vi "Write to file.vi"(8 "error in (no error)":errorcluster, 9 "Data Cluster":T4, 10 "Test Case":T5, 11 "Don't wait for stabilizatoin":bool) -> (0 "error out":errorcluster)   [LabVIEW 2013]
uses:
  Controls/Test Case.ctl
  Controls/Power Values.ctl
  <vilib>/addons/Electrical Power/Basic/Measurement/subVIs/basic_Power Value.ctl
  Controls/Stabilization.ctl
  <vilib>/addons/Electrical Power/Basic/NI_EP_Basic.lvlib
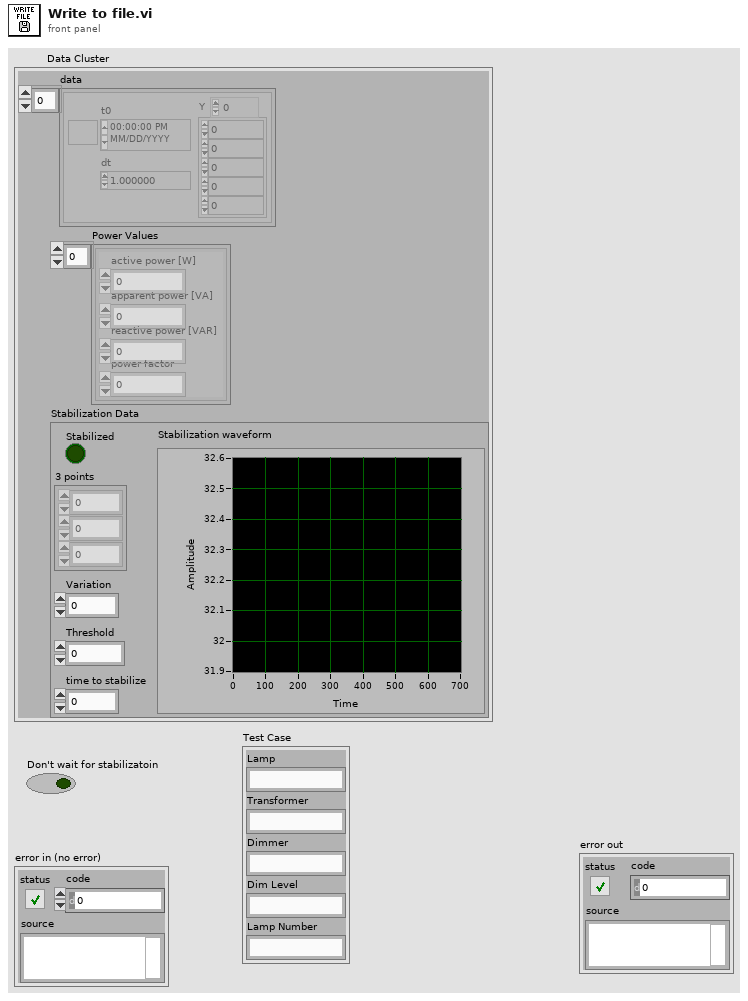
[diagram p1: front panel]
types:
  T1 = typedef "Power Values.ctl" = T2[]
  T2 = typedef "NI_EP_Basic.lvlib/basic_Power Value.ctl" = cluster{"active power [W]":dbl, "apparent power [VA]":dbl, "reactive power [VAR]":dbl, "power factor":dbl}
  T3 = typedef "Stabilization.ctl" = cluster{"Stabilization waveform":waveform(dbl), "Variation":dbl, "Stabilized":bool, "Threshold":dbl, "time to stabilize":dbl, "3 points":dbl[]}
  T4 = cluster{"data":waveform(dbl)[], "Power Values":T1, "Stabilization Data":T3}
  T5 = typedef "Test Case.ctl" = cluster{"Lamp":string, "Transformer":string, "Dimmer":string, "Dim Level":string, "Lamp Number":string}
  T6 = enum16{"open", "open or create", "create or replace", "create", "open (read-only)"}
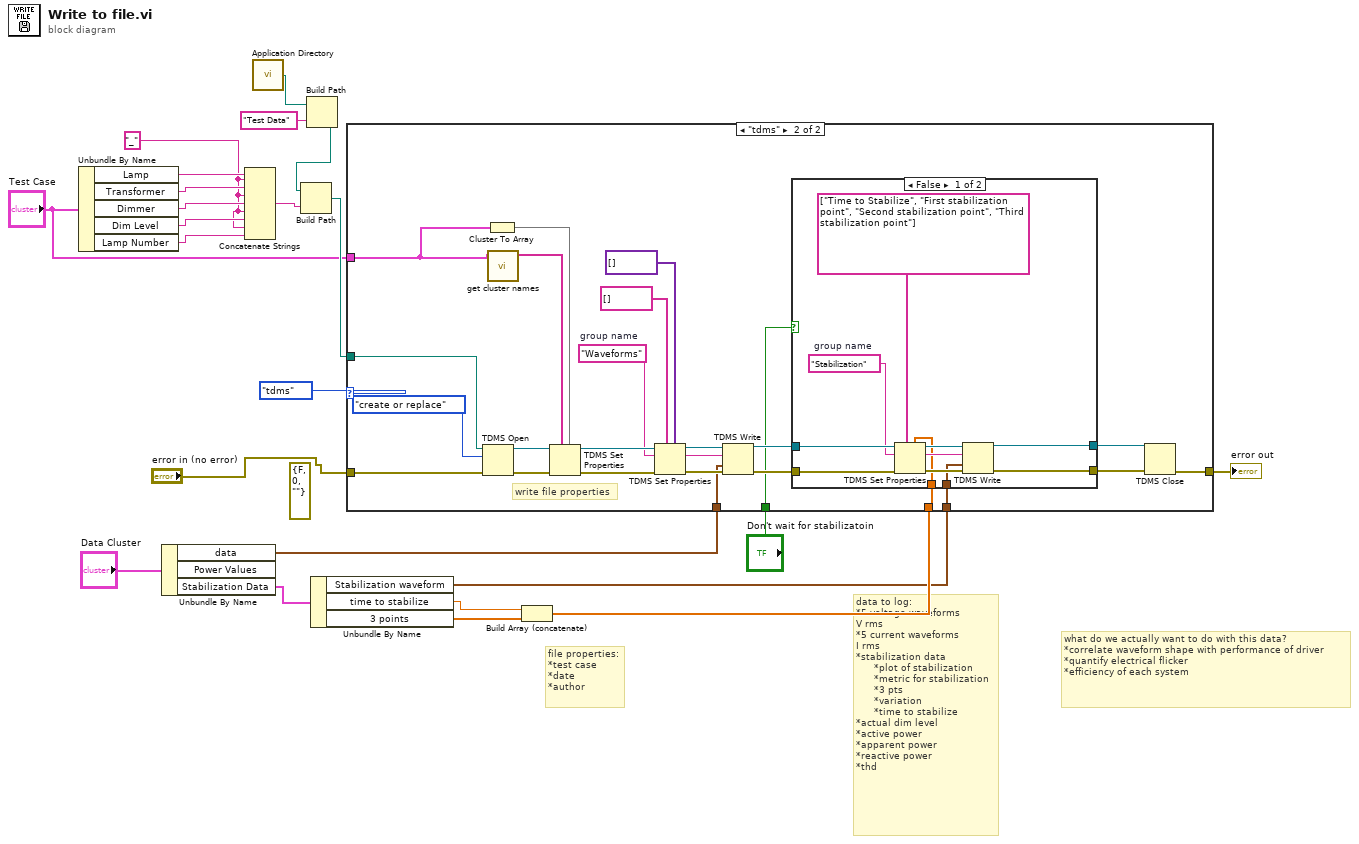
[diagram p0: block diagram]
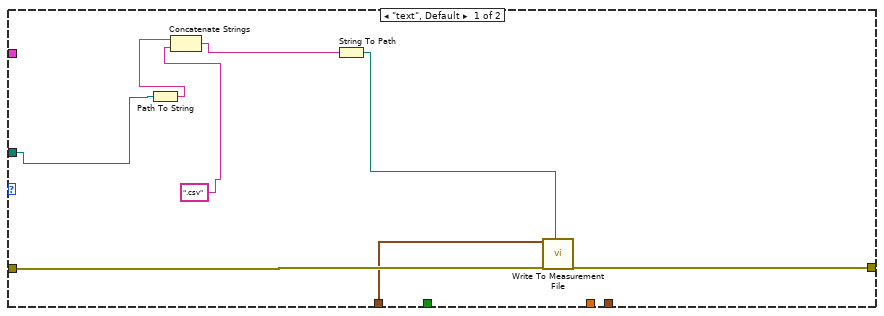
[diagram p2: hidden frame]
diagram:
  (unwired) errorcluster {"status"=FALSE, "code"=0, "source"=""} ("error in (no error)")
  w19 = "_"
  # "what do we actually want to do with this data?\n*correlate waveform shape with performance of driver\n*quantify electrical flicker\n*efficiency of each system"
  # "data to log:\n*5 voltage waveforms\nV rms\n*5 current waveforms\nI rms\n*stabilization data\n      *plot of stabilization\n      *metric for stabilization\n      *3 pts\n      *variation\n      *time to stabilize\n*actual dim level\n*active power\n*apparent power\n*reactive power\n*thd"
  # "file properties:\n*test case\n*date\n*author"
  n1 = Unbundle By Name("Test Case") -> ("Lamp"=w23:string, "Transformer"=w22:string, "Dimmer"=w21:string, "Dim Level"=w20:string, "Lamp Number"=w18:string)
  n2 = Unbundle By Name("Data Cluster") -> ("data"=w11:waveform(dbl)[], "Stabilization Data"=w10:T3)  [unwired: 1 out]
  n3 = Concatenate Strings(w23, w19, w22, w19, w21, w19, w20, w19, w18) -> (w17:string)
  n4 = call <vilib>:"Application Directory.vi"() -> ("Application Directory"=w3:path)
  n5 = Build Path(base path=w3, name or relative path="Test Data") -> (appended path=w2:path)
  n6 = Build Path(base path=w2, name or relative path=w17) -> (appended path=w16:path)
  n7 = Unbundle By Name(w10) -> ("Stabilization waveform"=w6:waveform(dbl), "time to stabilize"=w9:dbl, "3 points"=w8:dbl[])
  n8 = Build Array (concatenate)(w9, w8) -> (w7:dbl[])
  n9 = case shown="\"tdms\"" enum16{"tdms", "text"}."tdms" {
    tunnel: w16 -> [w28 w52]
    tunnel: "error in (no error)" -> [w31 w53]
    tunnel: [w30 w51] -> w14
    tunnel: w11 -> [w29 w41]
    tunnel: "Test Case" -> [_ w48]
    tunnel: w7 -> [_ w38]
    tunnel: w6 -> [_ w37]
    tunnel: "Don't wait for stabilizatoin" -> [_ w34]
    frame "text", Default {
      n10 = Path To String(path=w28) -> (string=w27:string)
      n11 = Concatenate Strings(w27, ".csv") -> (w25:string)
      n12 = String To Path(string=w25) -> (path=w24:path)
      n13 = call "Write To Measurement File"("Signals"=w29, "error in (no error)"=w31, "Filename"=w24) -> ("error out"=w30:errorcluster)  [unwired: 14 in, 2 out]
    }
    frame "tdms" {
      w45 = "Waveforms"  # group name
      # "write file properties"
      n14 = TDMS Open(8:w53, 10:T6."create or replace" ("operation (0:open)"), 11:w52) -> (0:w56:errorcluster, 3:w54:refnum<k34>)  [unwired: 4 in]
      n15 = Cluster To Array(cluster=w48) -> (array=w50:string[])
      n16 = call "get cluster names.vi"("Variant"=w48) -> ("Data Labels Array"=w49:string[])  [unwired: 10 in]
      n17 = TDMS Set Properties(5:w50, 7:w49, 8:w56, 11:w54) -> (0:w46:errorcluster, 3:w47:refnum<k34>)  [unwired: 2 in, 2 out]
      n18 = TDMS Set Properties(5:variant[] [] ("property values"), 7:string[] [] ("property names"), 8:w46, 10:w45, 11:w47) -> (0:w43:errorcluster, 2:w42:string, 3:w44:refnum<k34>)  [unwired: 1 in, 1 out]
      n19 = TDMS Write(0:w44, 5:w42, 9:w41, 11:w43) -> (4:w39:refnum<k34>, 15:w40:errorcluster)  [unwired: 2 in, 2 out]
      n20 = case shown="False" w34 {
        tunnel: w40 -> [w64 w68]
        tunnel: w39 -> [w63 w69]
        tunnel: w38 -> [w61 _]
        tunnel: w37 -> [w59 _]
        tunnel: [w58 w69] -> w36
        tunnel: [w57 w68] -> w35
        frame False {
          w62 = "Stabilization"  # group name
          n21 = TDMS Set Properties(5:w61, 7:string[] ["Time to Stabilize", "First stabilization point", "Second stabilization point", "Third stabilization point"] ("property names"), 8:w64, 10:w62, 11:w63) -> (0:w66:errorcluster, 2:w67:string, 3:w65:refnum<k34>)  [unwired: 1 in, 1 out]
          n22 = TDMS Write(0:w65, 5:w67, 9:w59, 11:w66) -> (4:w58:refnum<k34>, 15:w57:errorcluster)  [unwired: 2 in, 2 out]
        }
        frame True {
        }
      }
      n23 = TDMS Close(8:w35, 11:w36) -> (0:w51:errorcluster)  [unwired: 1 out]
    }
  }
  "error out" <- w14
